vi "Add.vi"() -> ()   [LabVIEW 2024, in "TypedCircularBuffer.Tests.Units.lvlib"]
uses:
  TypedCircularBuffer.Tests.Units.lvlib
  <vilib>/addons/_JKI Toolkits/Caraya/classes/Assert/Assert.lvclass
  <vilib>/addons/_JKI Toolkits/Caraya/classes/Test/Test.lvclass
  TypedCircularBuffer.lvclass
  <vilib>/addons/_JKI Toolkits/Caraya/classes/Assert/Assert True.vi
  Type.ctl
panel:
  in  "expected":i32[](array[numeric])=[1, 2, 3, 4, 5, 6, 7, 8, 9, 10]
  out "Flushed Buffer":T1[](array[typedef])
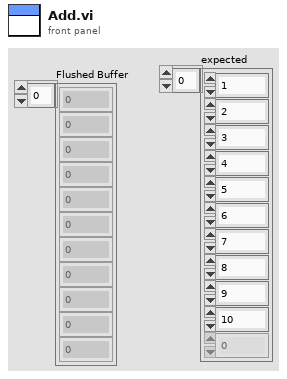
[diagram p1: front panel]
types:
  T1 = typedef "TypedCircularBuffer.lvclass/Type.ctl" = i32
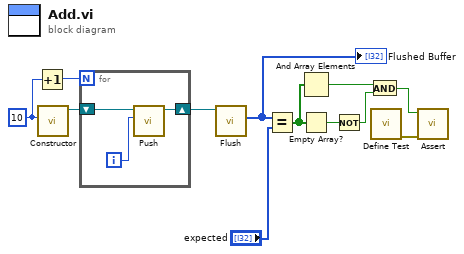
[diagram p0: block diagram]
diagram:
  w10 = u32 10 ("Capacity")
  n1 = Increment(x=w10) -> (x+1=w11:u32)
  n2 = call "Constructor.vi"("Capacity"=w10) -> ("TypedCircularBuffer out"=w12:refnum<class "TypedCircularBuffer.lvclass">)  [unwired: 10 in]
  n3 = for {
    N: w11 -> [_]
    shift-right: [w14] -> w9
    shift-left: w12 -> [w15]
    i -> [w13]
    n4 = call "Push.vi"("Element"=w13, "TypedCircularBuffer in"=w15) -> ("TypedCircularBuffer out"=w14:refnum<class "TypedCircularBuffer.lvclass">)  [unwired: 7 in, 2 out]
  }
  n5 = call "Flush.vi"("TypedCircularBuffer in"=w9) -> ("Flushed Buffer"=w2:T1[])  [unwired: 9 in, 1 out]
  "Flushed Buffer" <- w2
  n6 = Equal?(x=w2, y="expected") -> (x = y?=w5:bool[])
  n7 = And Array Elements(Boolean array=w5) -> (logical AND=w8:bool)
  n8 = Empty Array?(array=w5) -> (empty?=w7:bool)
  n9 = Not(x=w7) -> (.not. x?=w6:bool)
  n10 = And(x=w8, y=w6) -> (x .and. y?=w4:bool)
  n11 = call <vilib>:"Define Test.vi"() -> ("error out"=w3:errorcluster)  [unwired: 10 in, 1 out]
  n12 = call-poly <vilib>:"Assert.vi"("error in (no error)"=w3, "True?"=w4) -> ()  [unwired: 8 in, 2 out]
